vi "语音请求参数.vi"(10 "业务参数":T1, 11 "系统参数":T2) -> (3 "已排序的数组":T3[](array[typedef]))   [LabVIEW 2016]
uses:
  <vilib>/LVH/i3 OAuth/Controls/Name-Value Pair.ctl
  <vilib>/LVH/i3 OAuth/i3-oauth.lvlib
panel:
  out "数值":i32
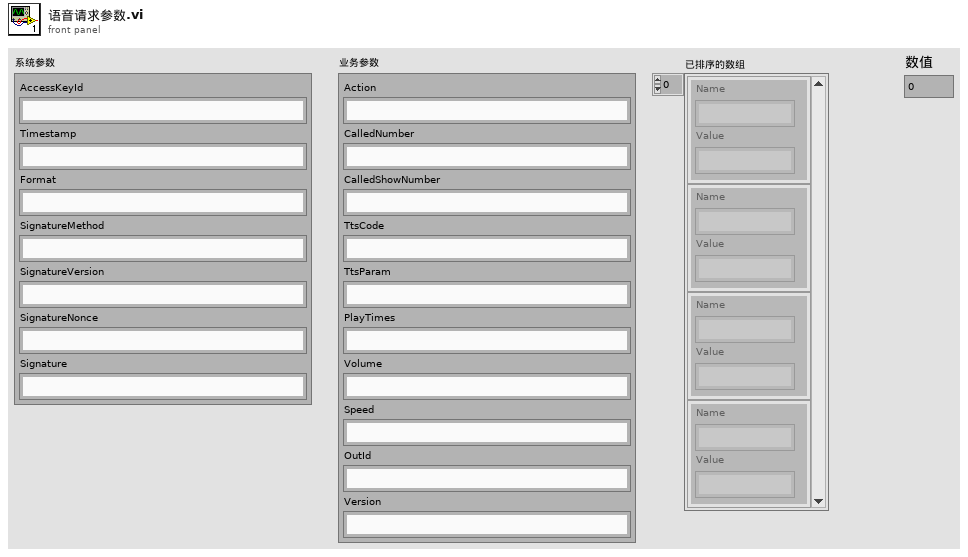
[diagram p1: front panel]
types:
  T1 = cluster{"Action":string, "CalledNumber":string, "CalledShowNumber":string, "TtsCode":string, "TtsParam":string, "PlayTimes":string, "Volume":string, "Speed":string, "OutId":string, "Version":string}
  T2 = cluster{"AccessKeyId":string, "Timestamp":string, "Format":string, "SignatureMethod":string, "SignatureVersion":string, "SignatureNonce":string, "Signature":string}
  T3 = typedef "i3-oauth.lvlib/Name-Value Pair.ctl" = cluster{"Name":string, "Value":string}
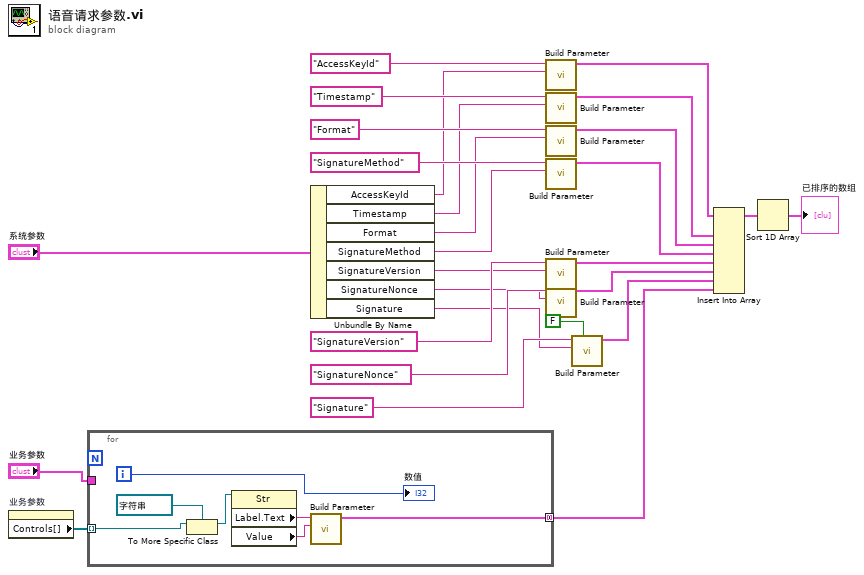
[diagram p0: block diagram]
diagram:
  n1 = property on="业务参数" class="Clust (严格)"() -> ("Controls[]"=w5:refnum<vi>[])  [unwired: 2 in, 2 out]
  n2 = for {
    tunnel: w5 -> [w34] mode=indexing
    tunnel: [w29] -> w4 mode=concatenating
    tunnel: "业务参数" -> [_]
    i -> [w32]
    n3 = To More Specific Class(target class=refnum<vi> refnum ("目标类"), reference=w34) -> (specific class reference=w33:refnum<vi>)  [unwired: 1 in, 1 out]
    n4 = property class="Str"(reference=w33) -> ("Label.Text"=w31:string, "Value"=w30:string)  [unwired: 1 in, 2 out]
    n5 = call <vilib>:"Build Parameter.vi"("Value"=w30, "Key"=w31) -> ("Parameter Array"=w29:T3[])  [unwired: 9 in]
    "数值" <- w32
  }
  n6 = Unbundle By Name("系统参数") -> ("AccessKeyId"=w12:string, "Timestamp"=w11:string, "Format"=w10:string, "SignatureMethod"=w9:string, "SignatureVersion"=w8:string, "SignatureNonce"=w7:string, "Signature"=w6:string)
  n7 = call <vilib>:"Build Parameter.vi"("Value"=w12, "Key"="AccessKeyId") -> ("Parameter Array"=w21:T3[])  [unwired: 9 in]
  n8 = call <vilib>:"Build Parameter.vi"("Value"=w11, "Key"="Timestamp") -> ("Parameter Array"=w20:T3[])  [unwired: 9 in]
  n9 = call <vilib>:"Build Parameter.vi"("Value"=w10, "Key"="Format") -> ("Parameter Array"=w19:T3[])  [unwired: 9 in]
  n10 = call <vilib>:"Build Parameter.vi"("Value"=w9, "Key"="SignatureMethod") -> ("Parameter Array"=w18:T3[])  [unwired: 9 in]
  n11 = call <vilib>:"Build Parameter.vi"("Value"=w8, "Key"="SignatureVersion") -> ("Parameter Array"=w17:T3[])  [unwired: 9 in]
  n12 = call <vilib>:"Build Parameter.vi"("Value"=w7, "Key"="SignatureNonce") -> ("Parameter Array"=w16:T3[])  [unwired: 9 in]
  n13 = call <vilib>:"Build Parameter.vi"("Return Parameter? (T)"=FALSE, "Value"=w6, "Key"="Signature") -> ("Parameter Array"=w15:T3[])  [unwired: 8 in]
  n14 = Insert Into Array(array=w21, new element #1=w20, new element #2=w19, new element #3=w18, new element #4=w17, new element #5=w16, new element #6=w15, new element #7=w4) -> (w3:T3[])  [unwired: 1 in]
  n15 = Sort 1D Array(array=w3) -> (sorted array=→"已排序的数组":T3[])
